vi "Get Encoder Wheel Values.vi"(8 "Reset encoder":bool, 10 "Wheel diameter (in)":dbl=6.0, 11 "refnum name":string="My Encoder RefNum") -> (0 "Encoder rate (deg/sec)":dbl, 1 "Distance (in)":dbl, 2 "Revolutions":dbl, 3 "Current angle (deg)":dbl(knob) scale=0.0..360.0, 4 "Direction moving":bool, 5 "Is moving":bool)   [LabVIEW 2014]
doc: "Handles a rotational encoder attached to a wheel and returns wheel direction, distance, velocity, state and angle."
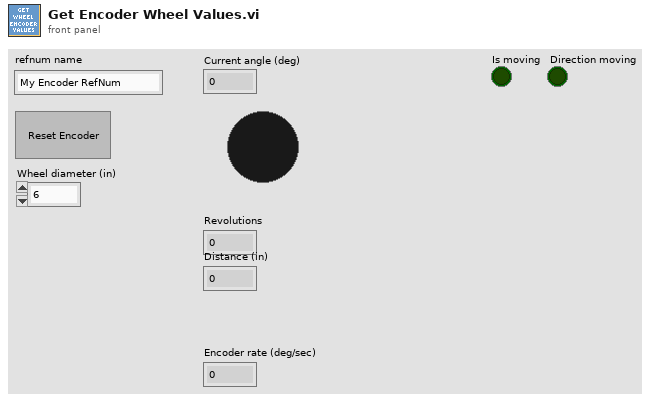
[diagram p1: front panel]
types:
  T1 = typedef "WPI_EncoderDevRef.ctl" = cluster{"DevStatus":errorcluster, "EncoderIndex":T2, "CounterIndex":T3, "DistancePerCount":dbl, "Decoding Type":T4}
  T2 = typedef "FPGA_EncoderIdx.ctl" = enum8{"Enc 0", "Enc 1", "Enc 2", "Enc 3", "Enc 4", "Enc 5", "Enc 6", "Enc 7", "Invalid"}
  T3 = typedef "FPGA_CounterCtrSystemIndex.ctl" = enum8{"Ctr 0", "Ctr 1", "Ctr 2", "Ctr 3", "Ctr 4", "Ctr 5", "Ctr 6", "Ctr 7", "Invalid"}
  T4 = typedef "WPI_EncoderType.ctl" = enum16{"1x", "2x", "4x"}
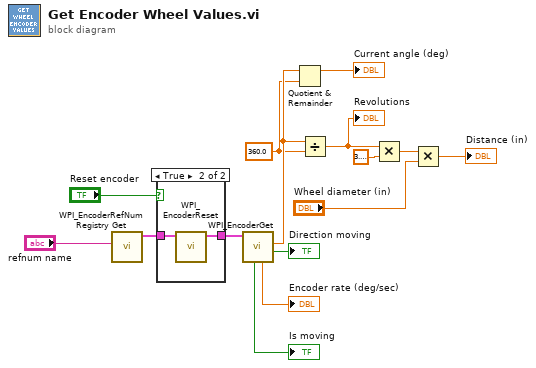
[diagram p0: block diagram]
diagram:
  w11 = 360.0 ("y")
  n1 = call <vilib>:"WPI_EncoderRefNum Registry Get.vi"("refnum name"="refnum name") -> ("EncoderDevRef"=w5:T1)  [unwired: 9 in, 1 out]
  n2 = case shown="True" "Reset encoder" {
    tunnel: w5 -> [w16 w18]
    tunnel: [w16 w17] -> w15
    frame False {
    }
    frame True {
      n3 = call <vilib>:"WPI_EncoderReset.vi"("EncoderDevRef"=w18) -> ("EncoderDevRef"=w17:T1)  [unwired: 1 in, 9 out]
    }
  }
  n4 = call <vilib>:"WPI_EncoderGet.vi"("EncoderDevRef"=w15) -> ("Direction"=→"Direction moving":bool, "Distance"=w12:dbl, "Rate"=→"Encoder rate (deg/sec)":dbl, "Stopped"=→"Is moving":bool)  [unwired: 1 in, 6 out]
  n5 = Quotient & Remainder(x=w12, y=w11) -> (x-y*floor(x/y)=→"Current angle (deg)":dbl)  [unwired: 1 out]
  n6 = Divide(x=w12, y=w11) -> (x/y=w10:dbl)
  "Revolutions" <- w10
  n7 = Multiply(x=w10, y=3.141592653589793) -> (x*y=w7:dbl)
  n8 = Multiply(x=w7, y="Wheel diameter (in)") -> (x*y=→"Distance (in)":dbl)
